vi "RPY_(SubVI).vi"(9 "XYZ":dbl[](array[numeric]) format="%0.2f", 10 "RPY angles":cluster{"roll":dbl, "pitch":dbl, "yaw":dbl}) -> (0 "POSE":dbl[](array[numeric]), 1 "Euler angles":T2, 2 "noa":cluster{T1, T1, T1}, 3 "Rotation matrix":dbl[][](array[numeric]))   [LabVIEW 2015]
uses:
  <vilib>/Analysis/Matrix/Datatypes/RealMatrix.ctl
  <vilib>/robotics/Kinematics/RotateX.vi
  <vilib>/robotics/Kinematics/RotateY.vi
  <vilib>/robotics/Kinematics/RotateZ.vi
  <vilib>/Analysis/baseanly.llb/A x B.vi
  <vilib>/Analysis/baseanly.llb/Real A x B.vi
  <vilib>/robotics/Kinematics/NI_Kinematics.lvlib
  <resource>/lvanlys.dll
  <vilib>/Analysis/Matrix/NI_Matrix.lvlib
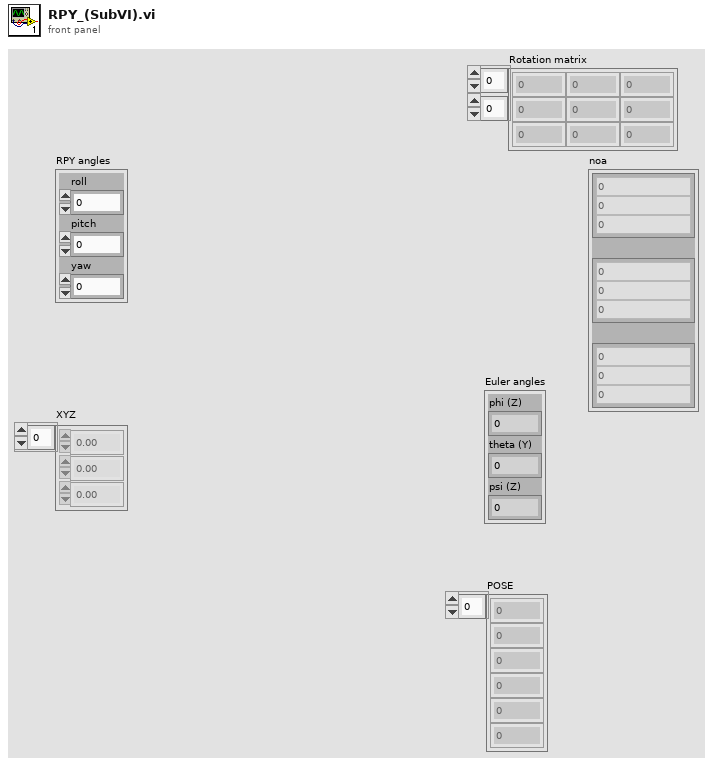
[diagram p1: front panel]
types:
  T1 = typedef "NI_Matrix.lvlib/RealMatrix.ctl" = dbl[][]
  T2 = cluster{"phi (Z)":dbl, "theta (Y)":dbl, "psi (Z)":dbl}
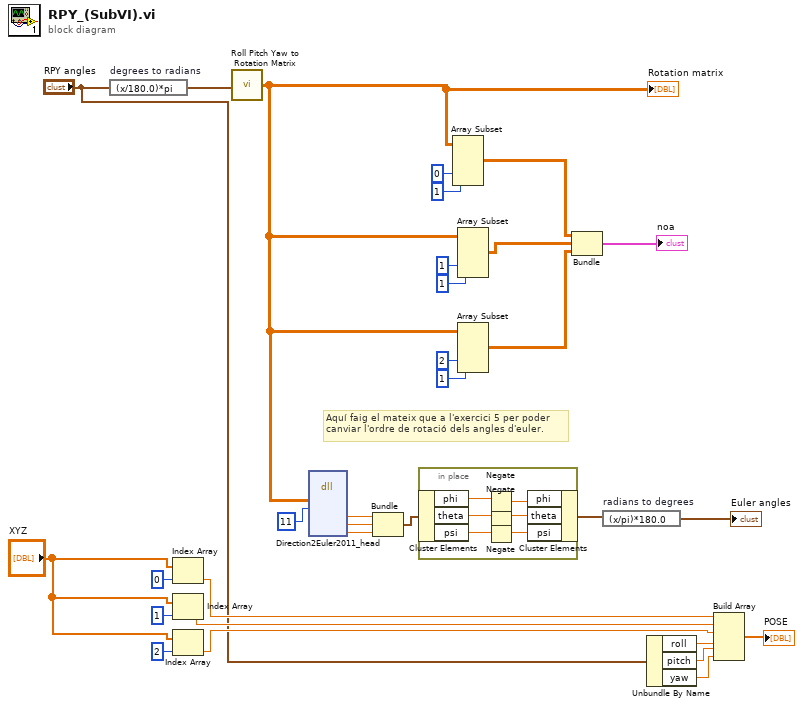
[diagram p0: block diagram]
diagram:
  # "Aquí faig el mateix que a l'exercici 5 per poder\ncanviar l'ordre de rotació dels angles d'euler."
  n1 = expression code="(x/180.0)*pi" "degrees to radians"("RPY angles") -> (w8:cluster{"roll":dbl, "pitch":dbl, "yaw":dbl})
  n2 = Index Array(array="XYZ", index=0) -> (element=w28:dbl)
  n3 = Index Array(array="XYZ", index=1) -> (element=w27:dbl)
  n4 = Index Array(array="XYZ", index=2) -> (element=w26:dbl)
  n5 = call <vilib>:"Roll Pitch Yaw to Rotation Matrix.vi"("angles"=w8) -> ("rotation matrix"=w4:T1)
  "Rotation matrix" <- w4
  n6 = dll-call lib="C:/Program Files (x86)/National Instruments/LabVIEW 2015/resource/lvanlys.*" fn="Direction2Euler2011_head"("direction"=w4, "rotateOrder"=11) -> ("phi"=w7:dbl, "theta"=w6:dbl, "psi"=w5:dbl)  [unwired: 9 in, 2 out]
  n7 = Bundle("phi"=w7, "theta"=w6, "psi"=w5) -> (w2:cluster{"phi":dbl, "theta":dbl, "psi":dbl})  [unwired: 1 in]
  n8 = in-place {
    n9 = in-place-cluster #1(w2) -> ("phi"=w37:dbl, "theta"=w35:dbl, "psi"=w33:dbl)
    n10 = Negate(x=w37) -> (-x=w36:dbl)
    n11 = Negate(x=w35) -> (-x=w34:dbl)
    n12 = Negate(x=w33) -> (-x=w32:dbl)
    n13 = in-place-cluster #1("phi"=w36, "theta"=w34, "psi"=w32) -> (w1:cluster{"phi":dbl, "theta":dbl, "psi":dbl})
  }
  n14 = Array Subset(array=w4, index (col)=0 ("index"), length (col)=1 ("length")) -> (w14:T1)  [unwired: 2 in]
  n15 = Array Subset(array=w4, index (col)=1 ("index"), length (col)=1 ("length")) -> (w13:T1)  [unwired: 2 in]
  n16 = Array Subset(array=w4, index (col)=2 ("index"), length (col)=1 ("length")) -> (w12:T1)  [unwired: 2 in]
  n17 = Bundle(w14, w13, w12) -> (→"noa":cluster{T1, T1, T1})  [unwired: 1 in]
  n18 = expression code="(x/pi)*180.0" "radians to degrees"(w1) -> (→"Euler angles":cluster{"phi":dbl, "theta":dbl, "psi":dbl})
  n19 = Unbundle By Name("RPY angles") -> ("roll"=w29:dbl, "pitch"=w30:dbl, "yaw"=w31:dbl)
  n20 = Build Array(w28, w27, w26, w29, w30, w31) -> (→"POSE":dbl[])
